vi "Read ZM_State.vi"(11 "valve_VCH_ZM_state in":refnum<class "valve_VCH_ZM_state.lvclass">) -> (2 "ZM_State_VCH":T1, 3 "valve_VCH_ZM_state out":refnum<class "valve_VCH_ZM_state.lvclass">)   [LabVIEW 2019, in "valve_VCH_ZM_state.lvclass"]
uses:
  valve_VCH_ZM_state.lvclass
  ctl/ZM_State_VCH.ctl
  valve_VCH_ZM_state.lvclass/valve_VCH_ZM_state.ctl
  Valves.lvlib
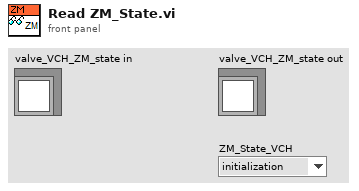
[diagram p1: front panel]
types:
  T1 = typedef "Valves.lvlib/ZM_State_VCH.ctl" = enum8{"initialization", "closed", "big_pause", "little_pause", "open", "close_cmd"}
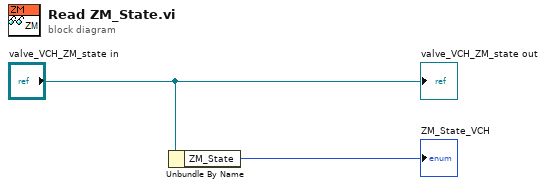
[diagram p0: block diagram]
diagram:
  n1 = Unbundle By Name("valve_VCH_ZM_state in") -> ("ZM_State"=→"ZM_State_VCH":T1)
  "valve_VCH_ZM_state out" <- "valve_VCH_ZM_state in"
